vi "XIPIN_ECC_2_0.vi"   [LabVIEW 2017]
doc: "ECC IP implements Hamming or HSIAO encoder decoder function for varying data widths\n------------------------------------\n<b>Need License</b> : No"
uses:
  <vilib>/rvi/XilinxIP/XIPIN_XNode/niFpgaXIPIN.xnode
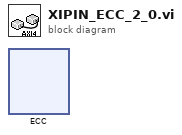
[diagram p0: block diagram]
diagram:
  n1 = xnode ("ECC")() -> ()
